vi "Chop One Bin.vi"(4 "tolerance":dbl=1e-16, 6 "variable output":string="y", 7 "variable input":string="x", 8 "error in (no error)":errorcluster, 9 "formula":string, 10 "chop?":bool, 11 "bin":cluster{"lower limit":dbl, "upper limit":dbl}) -> (0 "error out":errorcluster, 2 "Chop Out":bool[](array[boolean]), 3 "Bins Out":cluster{"lower limit":dbl, "upper limit":dbl}[](array[cluster]))   [LabVIEW 2020, in "NI_AALPro.lvlib"]
uses:
  <vilib>/Analysis/NI_AALPro.lvlib
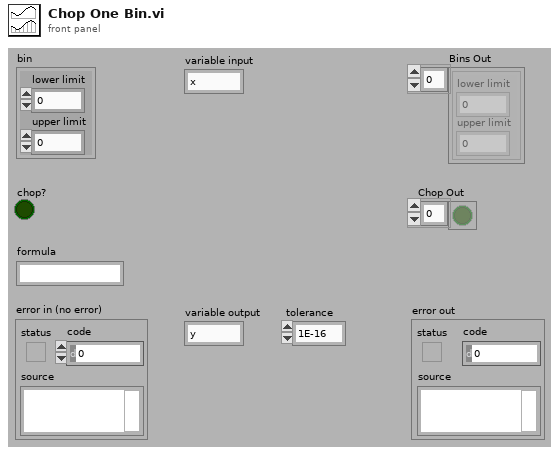
[diagram p1: front panel]
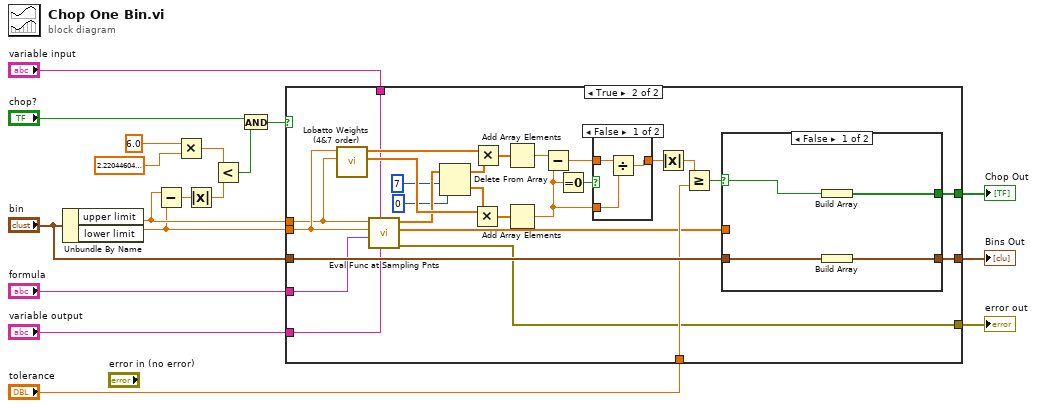
[diagram p0: block diagram]
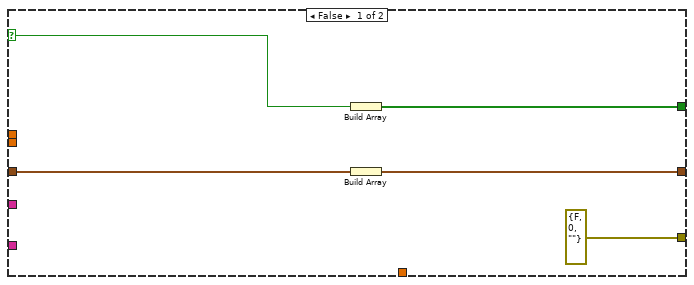
[diagram p2: hidden frame]
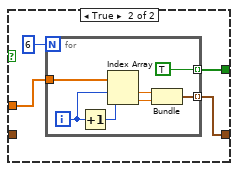
[diagram p4: hidden frame]
diagram:
  n1 = Unbundle By Name("bin") -> ("upper limit"=w13:dbl, "lower limit"=w12:dbl)
  n2 = Subtract(x=w13, y=w12) -> (x-y=w15:dbl)
  n3 = Multiply(x=6.0, y=2.220446049250313e-16 ("x^y")) -> (x*y=w6:dbl)
  n4 = Absolute Value(x=w15) -> (abs(x)=w7:dbl)
  n5 = Less?(x=w6, y=w7) -> (x < y?=w5:bool)
  n6 = And(x="chop?", y=w5) -> (x .and. y?=w11:bool)
  n7 = case shown="True" w11 {
    selector: w11 -> [w23 _]
    tunnel: [w20 w44] -> w18
    tunnel: [w22 w43] -> w17
    tunnel: "bin" -> [w21 w42]
    tunnel: w13 -> [_ w39]
    tunnel: w12 -> [_ w40]
    tunnel: "tolerance" -> [_ w41]
    tunnel: "variable input" -> [_ w32]
    tunnel: "variable output" -> [_ w30]
    tunnel: "formula" -> [_ w31]
    tunnel: [errorcluster {"status"=FALSE, "code"=0, "source"=""} ("error out") w29] -> w1
    frame False {
      n8 = Build Array(w23) -> (w22:bool[])
      n9 = Build Array(w21) -> (w20:cluster{"lower limit":dbl, "upper limit":dbl}[])
    }
    frame True {
      n10 = call <vilib>:"Lobatto Weights (4&7 order).vi"("lower limit"=w39, "upper limit"=w40) -> ("Weights (7-Order)"=w49:dbl[], "Weights (4-Order)"=w50:dbl[])  [unwired: 8 in]
      n11 = call <vilib>:"Eval Func at Sampling Pnts.vi"("variable output"=w30, "variable input"=w32, "formula"=w31, "lower limit"=w40, "upper limit"=w39) -> ("error out"=w29:errorcluster, "Sampling points (7-order)"=w38:dbl[], "Function Evaluations (7 and 4 pts)"=w28:dbl[])  [unwired: 4 in]
      n12 = Delete From Array(array=w28, length=7, index=0) -> (deleted portion=w24:dbl[], array with subset deleted=w25:dbl[])
      n13 = Multiply(x=w49, y=w24) -> (x*y=w47:dbl[])
      n14 = Multiply(x=w50, y=w25) -> (x*y=w48:dbl[])
      n15 = Add Array Elements(numeric array=w48) -> (sum=w46:dbl)
      n16 = Add Array Elements(numeric array=w47) -> (sum=w35:dbl)
      n17 = Subtract(x=w46, y=w35) -> (x-y=w36:dbl)
      n18 = Equal To 0?(x=w35) -> (x = 0?=w37:bool)
      n19 = case shown="False" w37 {
        tunnel: w36 -> [w53 w54]
        tunnel: w35 -> [w52 _]
        tunnel: [w51 w54] -> w34
        frame False {
          n20 = Divide(x=w53, y=w52) -> (x/y=w51:dbl)
        }
        frame True {
        }
      }
      n21 = Absolute Value(x=w34) -> (abs(x)=w33:dbl)
      n22 = Greater Or Equal?(x=w33, y=w41) -> (x >= y?=w45:bool)
      n23 = case shown="False" w45 {
        selector: w45 -> [w56 _]
        tunnel: w38 -> [_ w61]
        tunnel: [w57 w60] -> w44
        tunnel: w42 -> [w58 _]
        tunnel: [w55 w59] -> w43
        frame False {
          n24 = Build Array(w56) -> (w55:bool[])
          n25 = Build Array(w58) -> (w57:cluster{"lower limit":dbl, "upper limit":dbl}[])
        }
        frame True {
          n26 = for {
            N: 6 -> [_]
            tunnel: w61 -> [w69]
            tunnel: [w64] -> w60 mode=indexing
            tunnel: [TRUE] -> w59 mode=indexing
            i -> [w68]
            n27 = Increment(x=w68) -> (x+1=w67:i32)
            n28 = Index Array(array=w69, index #1=w68, index #2=w67) -> (element #1=w65:dbl, element #2=w66:dbl)
            n29 = Bundle(w65, w66) -> (w64:cluster{dbl, dbl})  [unwired: 1 in]
          }
        }
      }
    }
  }
  "Bins Out" <- w18
  "Chop Out" <- w17
  "error out" <- w1
